vi "LSX Get Encoder Position.vi"(8 "error in (no error)":errorcluster, 10 "pbValue":i32, 11 "lLSID":i32) -> (0 "error out":errorcluster, 2 "pbValue out":i32, 3 "function return":i32)   [LabVIEW 2018, in "Tango.lvlib"]
doc: "TANGOAPI int TANGOCALL LSX_GetEncoderPosition (int lLSID, BOOL *pbValue);"
uses:
  Tango.lvlib
  SubVIs/Tango_DLL.dll
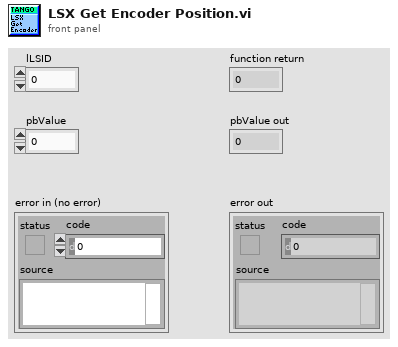
[diagram p1: front panel]
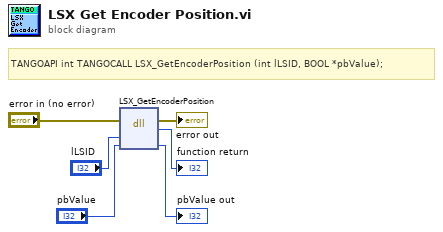
[diagram p0: block diagram]
diagram:
  # "TANGOAPI int TANGOCALL LSX_GetEncoderPosition (int lLSID, BOOL *pbValue);"
  n1 = dll-call lib="C:/Users/Familie/Documents/LabviewIX81/lib/TANGO Stage/SubVIs/Tango_DLL.*" fn="LSX_GetEncoderPosition"(error in="error in (no error)", "lLSID"="lLSID", "pbValue"="pbValue") -> (error out=→"error out":errorcluster, →"function return":i32, "pbValue"=→"pbValue out":i32)  [unwired: 3 in, 1 out]
